vi "trackGlobVarWrite.vi"(0 "dacStepSize18Bit":i32, 1 "dacStartRegister18Bit":i32, 2 "nOfSteps":i32, 3 "nOfScans":i32, 4 "invertScan":bool, 8 "VoltOrScaler?":bool, 9 "waitForKepco(25nsTicks)":u16, 11 "waitAfterReset(25nsTicks)":u16) -> ()   [LabVIEW 2014]
uses:
  <vilib>/rvi/Emulation/niFpgaSctlEmulationGetInTimedLoop.vi
  trackGlobVar.vi
  <vilib>/rvi/Emulation/niFpgaProcessEmulError.vi
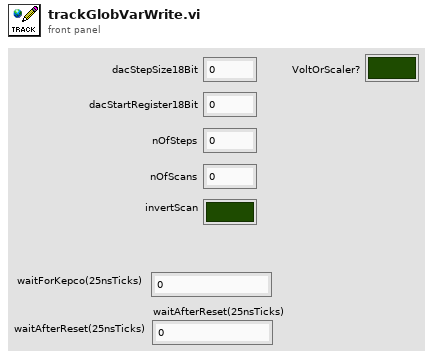
[diagram p1: front panel]
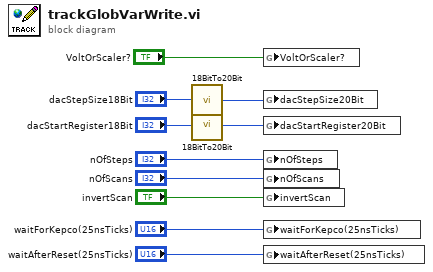
[diagram p0: block diagram]
diagram:
  n1 = call "18BitTo20Bit.vi"("18Bit"="dacStepSize18Bit") -> ("20Bit"=w3:i32)  [unwired: 4 in]
  n2 = call "18BitTo20Bit.vi"("18Bit"="dacStartRegister18Bit") -> ("20Bit"=w1:i32)  [unwired: 4 in]
  n3 = global write "trackGlobVar.vi" "VoltOrScaler?"("VoltOrScaler?") -> ()
  n4 = global write "trackGlobVar.vi" "dacStepSize20Bit"(w3) -> ()
  n5 = global write "trackGlobVar.vi" "dacStartRegister20Bit"(w1) -> ()
  n6 = global write "trackGlobVar.vi" "nOfSteps"("nOfSteps") -> ()
  n7 = global write "trackGlobVar.vi" "nOfScans"("nOfScans") -> ()
  n8 = global write "trackGlobVar.vi" "invertScan"("invertScan") -> ()
  n9 = global write "trackGlobVar.vi" "waitForKepco(25nsTicks)"("waitForKepco(25nsTicks)") -> ()
  n10 = global write "trackGlobVar.vi" "waitAfterReset(25nsTicks)"("waitAfterReset(25nsTicks)") -> ()
